vi "Close Test.vi"(8 "error in (no error)":errorcluster, 11 "Test Manager in":refnum<class "Basic Test Manager.lvclass">) -> (0 "error out":errorcluster, 3 "Test Manager out":refnum<class "Basic Test Manager.lvclass">)   [LabVIEW 2013, in "Caraya.lvlib" / "Basic Test Manager.lvclass"]
uses:
  Basic Test Manager.lvclass
  Test Result/Test Event Data.ctl
  Basic Test Manager.lvclass/Basic Test Manager.ctl
  Test Result/Test Result.lvclass
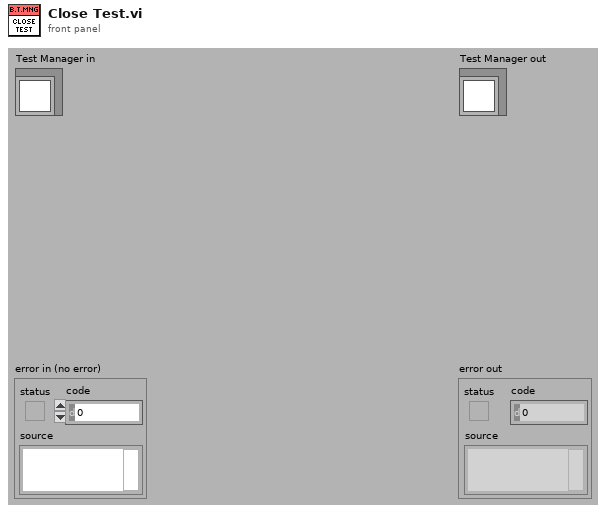
[diagram p1: front panel]
types:
  T1 = typedef "Caraya.lvlib/Test Result.lvclass/Test Event Data.ctl" = cluster{"Label":string, "Argument":variant}
  T2 = typedef "Caraya.lvlib/Test Result.lvclass/Test Event.ctl" = refnum<user-event>
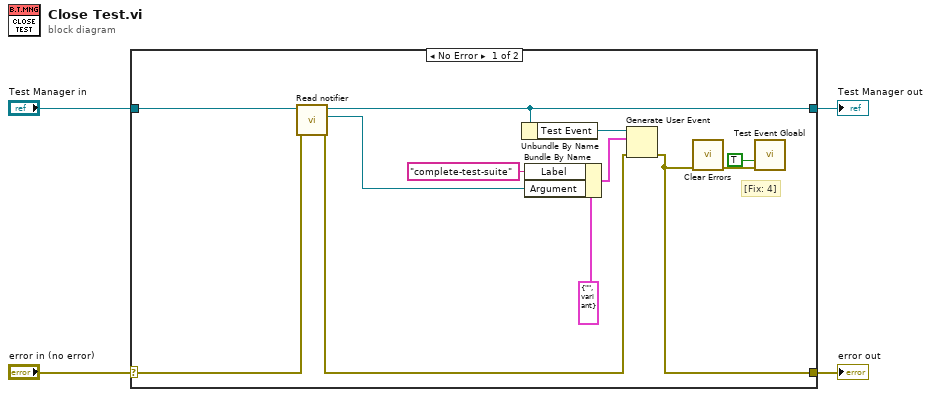
[diagram p0: block diagram]
diagram:
  n1 = case shown="No Error" "error in (no error)" {
    selector: "error in (no error)" -> [w6 w18]
    tunnel: [w12 w18] -> w3
    tunnel: [w7 w17] -> w1
    tunnel: "Test Manager in" -> [w8 w17]
    frame No Error {
      # "[Fix: 4]"
      n2 = call "Read notifier.vi"("error in (no error)"=w6, "Basic Test Manager in"=w8) -> ("error out"=w5:errorcluster, "notifier"=w9:refnum<notifier>, "Basic Test Manager out"=w7:refnum<class "Basic Test Manager.lvclass">)  [unwired: 7 in]
      n3 = Unbundle By Name(w7) -> ("Test Event"=w16:T2)
      n4 = Bundle By Name(cluster=T1 {"Label"="", "Argument"=variant} ("event data"), "Label"="complete-test-suite" ("Message"), "Argument"=w9) -> (w14:T1)
      n5 = Generate User Event(user event=w16, event data cluster=w14, error in=w5) -> (error out=w12:errorcluster)  [unwired: 1 in, 1 out]
      n6 = call <vilib>:"Clear Errors.vi"("error in (no error)"=w12) -> ("error out"=w11:errorcluster)  [unwired: 6 in]
      n7 = call "Test Event Gloabl.vi"("error in (no error)"=w11, "Clear (F)"=TRUE) -> ()  [unwired: 6 in, 4 out]
    }
    frame Error {
    }
  }
  "error out" <- w3
  "Test Manager out" <- w1
